vi "Global 1.vi"() -> ()   [LabVIEW 2017]
panel:
  in  "LastCount":dbl
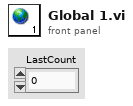
[diagram p1: front panel]
diagram:
